vi "Calculate center freq-core.vi"(7 "UI wavelength (nm)":dbl=920.0, 9 "AOL centre frequency (MHz)":dbl=39.0, 11 "AOL wavelength (nm)":dbl=800.0) -> (2 "Centre frequency (MHz)":dbl=39.0)   [LabVIEW 2017]
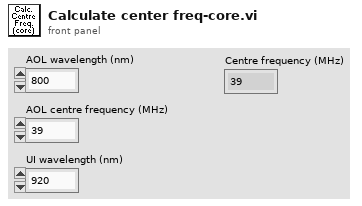
[diagram p1: front panel]
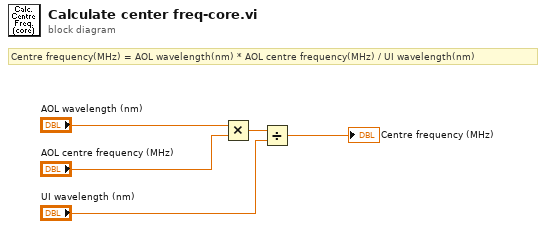
[diagram p0: block diagram]
diagram:
  # "Centre frequency(MHz) = AOL wavelength(nm) * AOL centre frequency(MHz) / UI wavelength(nm)"
  n1 = Multiply(x="AOL wavelength (nm)", y="AOL centre frequency (MHz)") -> (x*y=w3:dbl)
  n2 = Divide(x=w3, y="UI wavelength (nm)") -> (x/y=→"Centre frequency (MHz)":dbl)
